vi "Read (Single Response).vi"(8 "error in (no error)":errorcluster, 11 "VISA resource name":refnum<visa-resource-name>) -> (0 "error out":errorcluster, 1 "Response Bundle":T1, 2 "Response":string, 3 "VISA resource name out":refnum<visa-resource-name>, 4 "Message ID":i32)   [LabVIEW 2015, in "Zaber A Series.lvlib"]
doc: "Reads a single response from the Serial buffer. The complete string is returned on the Response output, and the details of the format of the response are described here: http://www.zaber.com/wiki/Manuals/ASCII_Protocol_Manual#Replies. This VI also validates checksums if present, combines multi-packet messages if needed, parses the message, bundles the components, and returns the bundle on the Response Bundle pin. \n\nThe Response Bundle is designed to extract data from Replies only. Info and Alert type responses will not make sense in the Bundle and should be read with just the Response output. By default the only Info or Alert type responses you can expect directly follow 'help' commands. \n\nThis VI requires that the Initialize VI has been called with the same serial port. \n\nThe Data string of the response is checked for rejection responses and if any are detected will send a warning or error on the error out. The possible warnings and errors are:\n\n-1074000003 - BADCHECKSUM - The checksum of a reply message indicates a transmission error.\n-1074000004 - BADFLAGS - The reply flags field of a response was not one of the legal values.\n-1074000005 - BADPACKET - A message did not start with one of the legal marker characters.\n-1074000006 - BADSEQUENCE - A multi-packet message could not be combined.\n1073481729 - BADCHECKSUM - The checksum provided in the command message was incorrect.\n1073481730 - BADCOMMAND - The command or setting is incorrect or invalid.\n1073481731 - BADDATA - The data provided in the command is incorrect or out of range.\n1073481732 - STATUSBUSY - The device cannot be parked, nor can certain settings be changed, because it is currently busy.\n1073481733 - DEVICEONLY - An axis number was specified when trying to execute a device only command.\n1073481734 - PARKED - The device cannot move because it is currently parked.\n1073481735 - AGAIN - The stream queue is full. The command should be resent until AGAIN is not received. \n1073481736 - BADMESSAGEID - A message ID was provided, but was not either -- or a number from 0 to 99.\n1073481737 - BADAXIS - The command was sent with an axis number greater than the number of axes available.\n1073481738 - LOCKSTEP - An axis cannot be moved using normal motion commands because it is part of a lockstep group. You must use lockstep commands for motion or disable the lockstep group first.\n1073481739 - FULL - The device has run out of permanent storage and cannot accept the command. Occurs when storing to a stream buffer or when saving commands to joystick keys.\n1073481740 - NOACCESS - The command or setting is not available at the current access level.\n\nNote: This VI is set to read 100 bytes at a time, but will terminate each read when it sees the new line character in order to return only one response. It's assumed that responses will be shorter than 100 characters. If your responses exceed this for any reason, adjust the constant to a higher number."
uses:
  Zaber A Series.lvlib
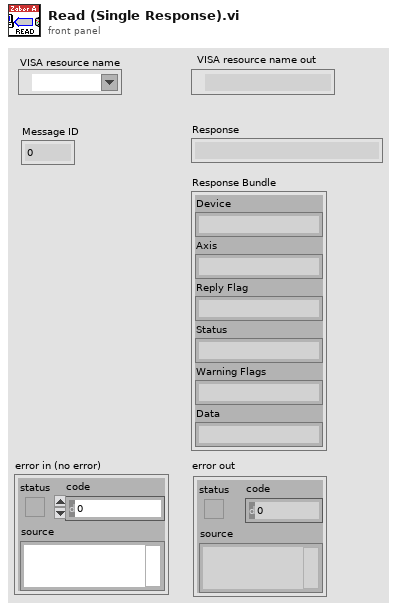
[diagram p1: front panel]
types:
  T1 = cluster{"Device":string, "Axis":string, "Reply Flag":string, "Status":string, "Warning Flags":string, "Data":string}
  T2 = cluster{string, string, string, string, string, "spreadsheet string":string}
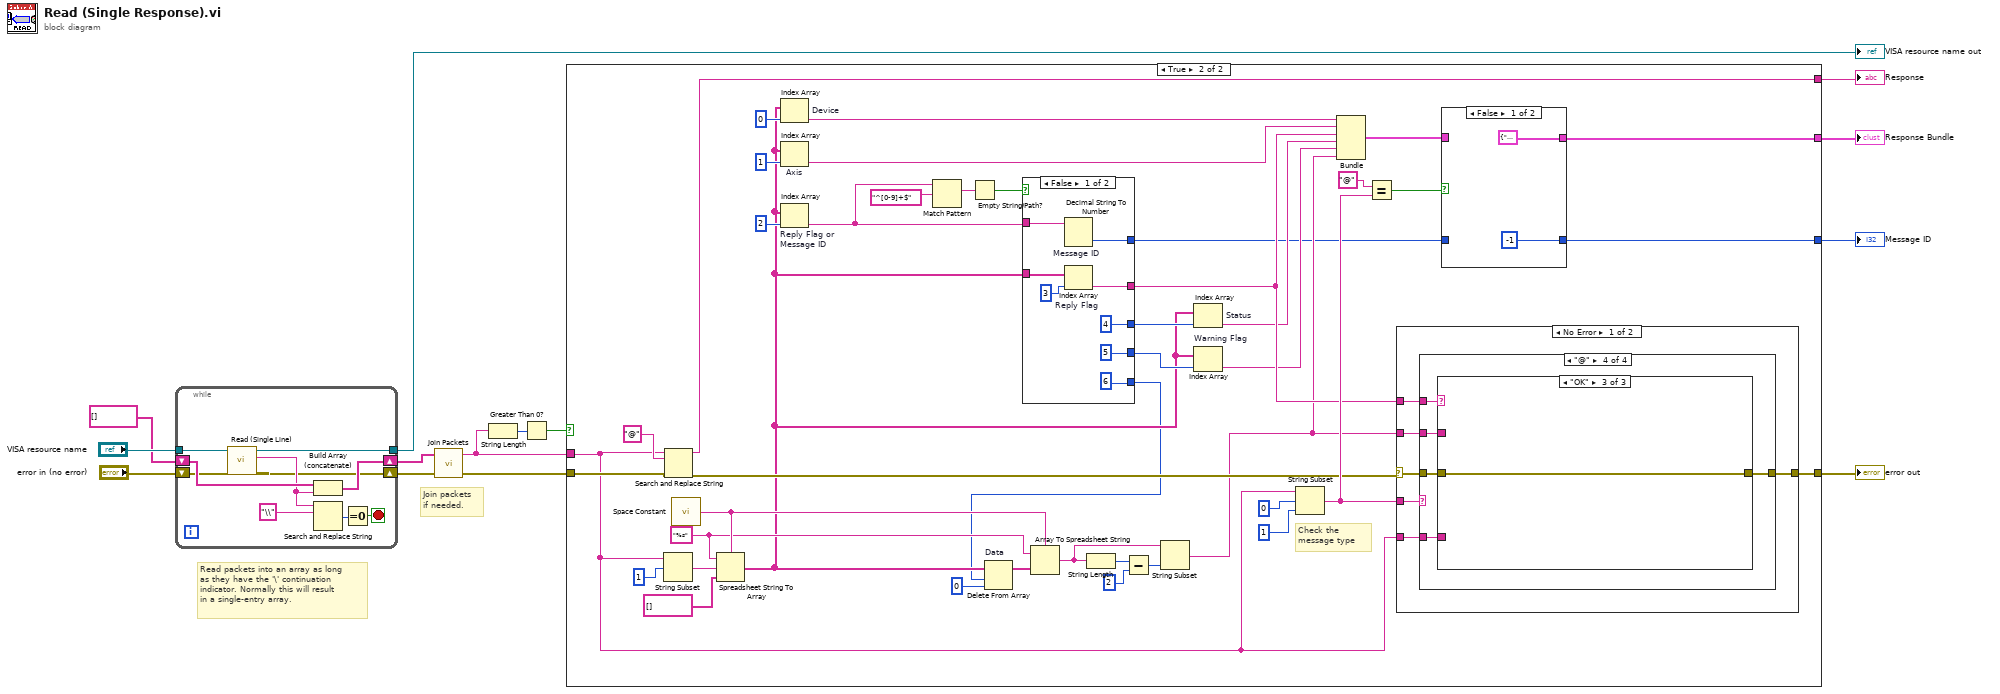
[diagram p0: block diagram]
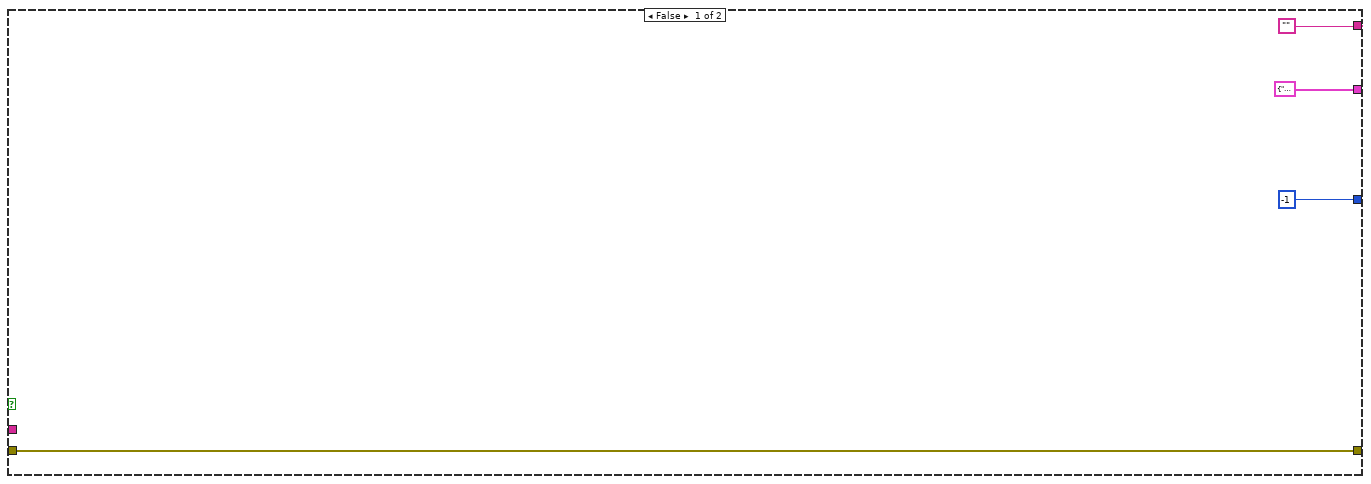
[diagram p2: hidden frame]
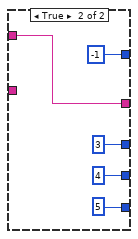
[diagram p3: hidden frame]
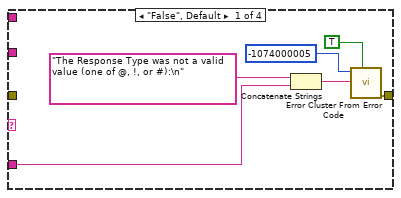
[diagram p5: hidden frame]
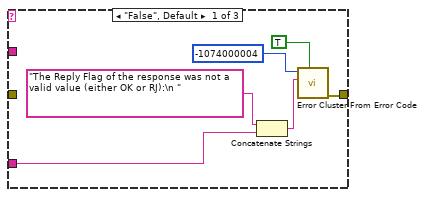
[diagram p8: hidden frame]
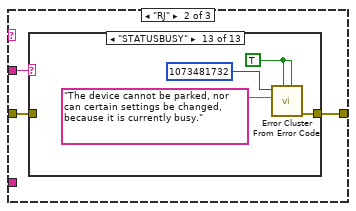
[diagram p9: hidden frame]
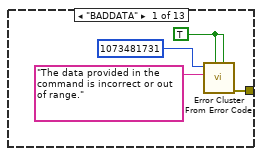
[diagram p10: hidden frame]
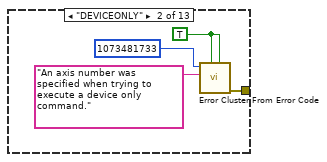
[diagram p11: hidden frame]
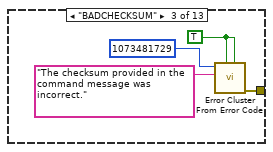
[diagram p12: hidden frame]
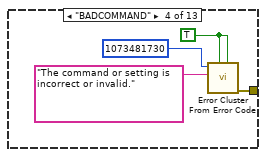
[diagram p13: hidden frame]
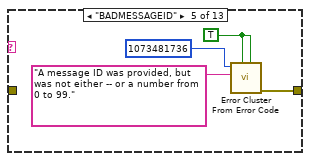
[diagram p14: hidden frame]
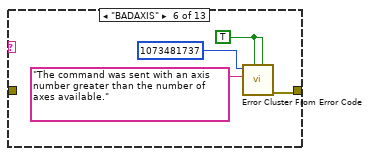
[diagram p15: hidden frame]
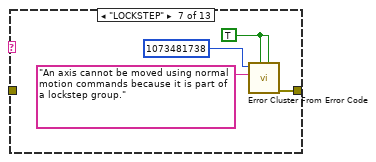
[diagram p16: hidden frame]
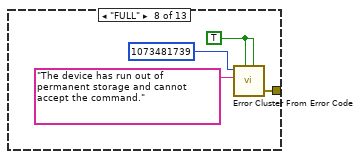
[diagram p17: hidden frame]
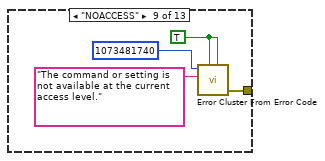
[diagram p18: hidden frame]
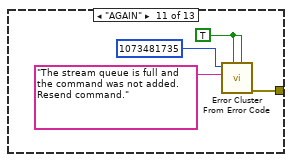
[diagram p20: hidden frame]
diagram:
  # "Join packets\nif needed."
  # "Read packets into an array as long\nas they have the '\\' continuation\nindicator. Normally this will result\nin a single-entry array."
  n1 = while {
    shift-right: [w16] -> w7
    shift-left: "error in (no error)" -> [w17]
    shift-right: [w21] -> w8
    shift-left: string[] [] -> [w20]
    tunnel: "VISA resource name" -> [w15]
    tunnel: [w19] -> w12
    stop <- w22 stop-if-true
    n2 = call "Read (Single Line).vi"("error in"=w17, "VISA resource name"=w15) -> ("error out"=w16:errorcluster, "Line"=w18:string, "VISA resource name 2"=w19:refnum<visa-resource-name>)  [unwired: 7 in]
    n3 = Build Array (concatenate)(w20, w18) -> (w21:string[])
    n4 = Search and Replace String(input string=w18, search string="\\") -> (number of replacements=w24:i32)  [unwired: 6 in, 3 out]
    n5 = Equal To 0?(x=w24) -> (x = 0?=w22:bool)
  }
  "VISA resource name out" <- w12
  n6 = call "Join Packets.vi"("error in (no error)"=w7, "Packets"=w8) -> ("error out"=w6:errorcluster, "Response"=w4:string)  [unwired: 2 in]
  n7 = String Length(string=w4) -> (length=w5:i32)
  n8 = Greater Than 0?(x=w5) -> (x > 0?=w3:bool)
  n9 = case shown="True" w3 {
    tunnel: [w27 w71] -> w11
    tunnel: [T1 {"Device"="", "Axis"="", "Reply Flag"="", "Status"="", "Warning Flags"="", "Data"=""} w57] -> w10
    tunnel: w4 -> [_ w33]
    tunnel: w6 -> [w27 w48]
    tunnel: ["" w46] -> w2
    tunnel: [-1 w30] -> w1
    frame False {
    }
    frame True {
      w61 = "%s" ("format string")
      # "Check the\nmessage type"
      n10 = String Subset(string=w33, offset (0)=1) -> (substring=w50:string)  [unwired: 1 in]
      n11 = Search and Replace String(input string=w33, search string="@" ("substring (\"\")"), error in=w48) -> (result string=w46:string, error out=w47:errorcluster)  [unwired: 5 in, 2 out]
      n12 = call <vilib>:"Space Constant.vi"() -> ("String"=w66:string)
      n13 = Spreadsheet String To Array(delimiter (Tab)=w66, format string=w61, spreadsheet string=w50, array type (2D Dbl)=string[] []) -> (array=w35:string[])
      n14 = Index Array "Device"(array=w35, index=0) -> (element=w69:string)
      n15 = Index Array "Axis"(array=w35, index=1) -> (element=w68:string)
      n16 = Index Array "Reply Flag or\nMessage ID"(array=w35, index=2) -> (element=w42:string)
      n17 = Match Pattern(string=w42, regular expression="^[0-9]+$") -> (match substring=w41:string)  [unwired: 1 in, 3 out]
      n18 = Empty String/Path?(string/path=w41) -> (empty?=w44:bool)
      n19 = case shown="False" w44 {
        tunnel: [w75 w84] -> w43
        tunnel: w42 -> [w74 w84]
        tunnel: [4 ("index") 3 ("index")] -> w38
        tunnel: [5 ("index") 4 ("index")] -> w37
        tunnel: w35 -> [w76 _]
        tunnel: [w73 -1] -> w29
        tunnel: [6 ("length") 5] -> w34
        frame False {
          n20 = Decimal String To Number "Message ID"(string=w74) -> (number=w73:i32)  [unwired: 2 in, 1 out]
          n21 = Index Array "Reply Flag"(array=w76, index=3) -> (element=w75:string)
        }
        frame True {
        }
      }
      n22 = Delete From Array "Data"(array=w35, length=w34, index=0) -> (array with subset deleted=w67:string[])  [unwired: 1 out]
      n23 = Array To Spreadsheet String(delimiter (Tab)=w66, array=w67, 3:w61) -> (spreadsheet string=w32:string)
      n24 = String Length(string=w32) -> (length=w36:i32)
      n25 = Subtract(x=w36, y=2) -> (x-y=w52:i32)
      n26 = String Subset(string=w32, length (rest)=w52) -> (substring=w31:string)  [unwired: 1 in]
      n27 = Index Array "Status"(array=w35, index=w38) -> (element=w40:string)
      n28 = Index Array "Warning Flag"(array=w35, index=w37) -> (element=w39:string)
      n29 = String Subset(string=w33, offset (0)=0, length (rest)=1 ("length (rest)")) -> (substring=w56:string)
      n30 = Bundle(w69, w68, w43, w40, w39, "spreadsheet string"=w31) -> (w58:T2)  [unwired: 1 in]
      n31 = Equal?(x="@", y=w56) -> (x = y?=w54:bool)
      n32 = case shown="No Error" w47 {
        selector: w47 -> [w92 w167]
        tunnel: [w94 w167] -> w71
        tunnel: w31 -> [w93 _]
        tunnel: w56 -> [w91 _]
        tunnel: w43 -> [w90 _]
        tunnel: w33 -> [w89 _]
        frame No Error {
          n33 = case shown="\"@\"" w91 {
            tunnel: [w98 w101 w102 w107] -> w94
            tunnel: w93 -> [_ _ _ w106]
            tunnel: w92 -> [_ w101 w102 w105]
            tunnel: w90 -> [_ _ _ w104]
            tunnel: w89 -> [w95 _ _ w103]
            frame "False", Default {
              n34 = Concatenate Strings("The Response Type was not a valid value (one of @, !, or #):\n" ("error message (\"\")"), w95) -> (w97:string)
              n35 = call <vilib>:"Error Cluster From Error Code.vi"("show call chain? (False)"=TRUE, "error message (\"\")"=w97, "error code (0)"=-1074000005) -> ("error out"=w98:errorcluster)  [unwired: 6 in]
            }
            frame "!" {
            }
            frame "#" {
            }
            frame "@" {
              n36 = case shown="\"OK\"" w104 {
                tunnel: [w111 w116 w166] -> w107
                tunnel: w106 -> [_ w115 _]
                tunnel: w105 -> [_ w114 w166]
                tunnel: w103 -> [w110 _ _]
                frame "False", Default {
                  n37 = Concatenate Strings("The Reply Flag of the response was not a valid value (either OK or RJ):\n " ("error message (\"\")"), w110) -> (w108:string)
                  n38 = call <vilib>:"Error Cluster From Error Code.vi"("show call chain? (False)"=TRUE, "error message (\"\")"=w108, "error code (0)"=-1074000004) -> ("error out"=w111:errorcluster)  [unwired: 6 in]
                }
                frame "RJ" {
                  n39 = case shown="\"STATUSBUSY\"" w115 {
                    tunnel: [w117 w123 w125 w129 w133 w137 w141 w145 w149 w153 w154 w159 w163] -> w116
                    tunnel: w114 -> [_ _ _ _ _ _ _ _ _ w153 _ _ _]
                    frame "BADDATA" {
                      w120 = TRUE
                      n40 = call <vilib>:"Error Cluster From Error Code.vi"("is warning? (False)"=w120, "show call chain? (False)"=w120, "error message (\"\")"="The data provided in the command is incorrect or out of range." ("error message (\"\")"), "error code (0)"=1073481731) -> ("error out"=w117:errorcluster)  [unwired: 5 in]
                    }
                    frame "DEVICEONLY" {
                      w124 = TRUE
                      n41 = call <vilib>:"Error Cluster From Error Code.vi"("is warning? (False)"=w124, "show call chain? (False)"=w124, "error message (\"\")"="An axis number was specified when trying to execute a device only command." ("error message (\"\")"), "error code (0)"=1073481733) -> ("error out"=w123:errorcluster)  [unwired: 5 in]
                    }
                    frame "BADCHECKSUM" {
                      w128 = TRUE
                      n42 = call <vilib>:"Error Cluster From Error Code.vi"("is warning? (False)"=w128, "show call chain? (False)"=w128, "error message (\"\")"="The checksum provided in the command message was incorrect." ("error message (\"\")"), "error code (0)"=1073481729) -> ("error out"=w125:errorcluster)  [unwired: 5 in]
                    }
                    frame "BADCOMMAND" {
                      w132 = TRUE
                      n43 = call <vilib>:"Error Cluster From Error Code.vi"("is warning? (False)"=w132, "show call chain? (False)"=w132, "error message (\"\")"="The command or setting is incorrect or invalid." ("error message (\"\")"), "error code (0)"=1073481730) -> ("error out"=w129:errorcluster)  [unwired: 5 in]
                    }
                    frame "BADMESSAGEID" {
                      w136 = TRUE
                      n44 = call <vilib>:"Error Cluster From Error Code.vi"("is warning? (False)"=w136, "show call chain? (False)"=w136, "error message (\"\")"="A message ID was provided, but was not either -- or a number from 0 to 99." ("error message (\"\")"), "error code (0)"=1073481736) -> ("error out"=w133:errorcluster)  [unwired: 5 in]
                    }
                    frame "BADAXIS" {
                      w138 = TRUE
                      n45 = call <vilib>:"Error Cluster From Error Code.vi"("is warning? (False)"=w138, "show call chain? (False)"=w138, "error message (\"\")"="The command was sent with an axis number greater than the number of axes available." ("error message (\"\")"), "error code (0)"=1073481737) -> ("error out"=w137:errorcluster)  [unwired: 5 in]
                    }
                    frame "LOCKSTEP" {
                      w144 = TRUE
                      n46 = call <vilib>:"Error Cluster From Error Code.vi"("is warning? (False)"=w144, "show call chain? (False)"=w144, "error message (\"\")"="An axis cannot be moved using normal motion commands because it is part of a lockstep group." ("error message (\"\")"), "error code (0)"=1073481738) -> ("error out"=w141:errorcluster)  [unwired: 5 in]
                    }
                    frame "FULL" {
                      w146 = TRUE
                      n47 = call <vilib>:"Error Cluster From Error Code.vi"("is warning? (False)"=w146, "show call chain? (False)"=w146, "error message (\"\")"="The device has run out of permanent storage and cannot accept the command." ("error message (\"\")"), "error code (0)"=1073481739) -> ("error out"=w145:errorcluster)  [unwired: 5 in]
                    }
                    frame "NOACCESS" {
                      w152 = TRUE
                      n48 = call <vilib>:"Error Cluster From Error Code.vi"("is warning? (False)"=w152, "show call chain? (False)"=w152, "error message (\"\")"="The command or setting is not available at the current access level." ("error message (\"\")"), "error code (0)"=1073481740) -> ("error out"=w149:errorcluster)  [unwired: 5 in]
                    }
                    frame Default {
                    }
                    frame "AGAIN" {
                      w157 = TRUE
                      n49 = call <vilib>:"Error Cluster From Error Code.vi"("is warning? (False)"=w157, "show call chain? (False)"=w157, "error message (\"\")"="The stream queue is full and the command was not added. Resend command." ("error message (\"\")"), "error code (0)"=1073481735) -> ("error out"=w154:errorcluster)  [unwired: 5 in]
                    }
                    frame "PARKED" {
                      w161 = TRUE
                      n50 = call <vilib>:"Error Cluster From Error Code.vi"("is warning? (False)"=w161, "show call chain? (False)"=w161, "error message (\"\")"="The device cannot move because it is currently parked." ("error message (\"\")"), "error code (0)"=1073481734) -> ("error out"=w159:errorcluster)  [unwired: 5 in]
                    }
                    frame "STATUSBUSY" {
                      w165 = TRUE
                      n51 = call <vilib>:"Error Cluster From Error Code.vi"("is warning? (False)"=w165, "show call chain? (False)"=w165, "error message (\"\")"="The device cannot be parked, nor can certain settings be changed, because it is currently busy." ("error message (\"\")"), "error code (0)"=1073481732) -> ("error out"=w163:errorcluster)  [unwired: 5 in]
                    }
                  }
                }
                frame "OK" {
                }
              }
            }
          }
        }
        frame Error {
        }
      }
      n52 = case shown="False" w54 {
        tunnel: w58 -> [_ w88]
        tunnel: [T2 {"", "", "", "", "", "spreadsheet string"=""} ("output cluster") w88] -> w57
        tunnel: [-1 w87] -> w30
        tunnel: w29 -> [_ w87]
        frame False {
        }
        frame True {
        }
      }
    }
  }
  "error out" <- w11
  "Response" <- w2
  "Response Bundle" <- w10
  "Message ID" <- w1
